vi "Get Lifecycle State.vi"(8 "error in (no error)":errorcluster, 11 "Process In":refnum<class "Process.lvclass">) -> (0 "error out":errorcluster, 1 "In Process Loop?":bool, 2 "Lifecycle State":T1, 3 "Process Out":refnum<class "Process.lvclass">)   [LabVIEW 2020, in "Process.lvclass"]
doc: "Returns the current life cycle state of the process. The \"In Process Loop?\" flag indicates wether the VI is called from within the process loop of the class calling it."
uses:
  Process.lvclass
  TypeDefs/Lifecycle State.ctl
  Process.lvclass/Process.ctl
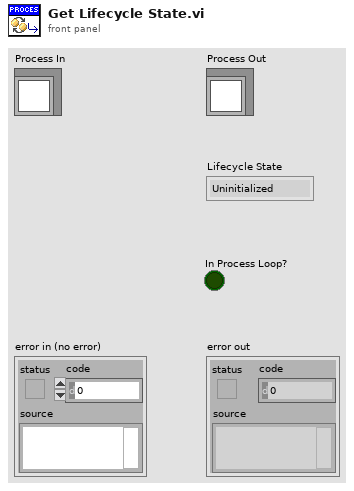
[diagram p1: front panel]
types:
  T1 = typedef "Process.lvclass/Lifecycle State.ctl" = enum16{"Uninitialized", "Initialized", "Started", "Running", "Stopped", "Finished"}
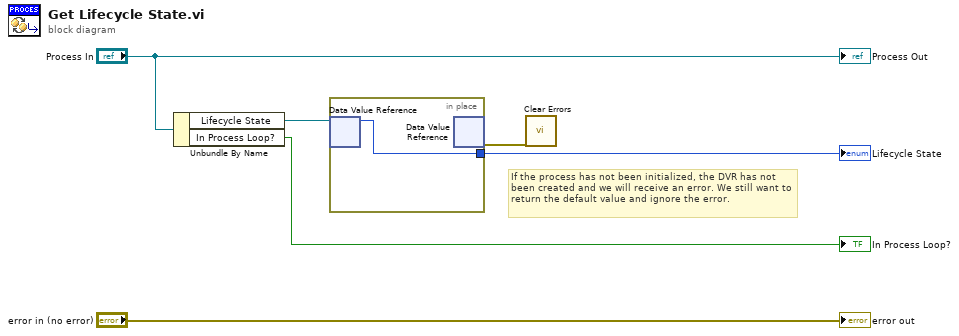
[diagram p0: block diagram]
diagram:
  # "If the process has not been initialized, the DVR has not been created and we will receive an error. We still want to return the default value and ignore the error."
  n1 = Unbundle By Name("Process In") -> ("Lifecycle State"=w5:refnum<data-value>, "In Process Loop?"=→"In Process Loop?":bool)
  n2 = in-place {
    in-place-border: [w7] -> w3
    n3 = in-place-dvr #1(w5) -> (w7:T1)  [unwired: 1 out]
    n4 = in-place-dvr #1() -> (w2:errorcluster)  [unwired: 1 in, 1 out]
  }
  "Lifecycle State" <- w3
  n5 = call <vilib>:"Clear Errors.vi"("error in (no error)"=w2) -> ()  [unwired: 5 in, 2 out]
  "error out" <- "error in (no error)"
  "Process Out" <- "Process In"
